vi "仿真全局变量.vi"() -> ()   [LabVIEW 2016, in "仿真数据.lvlib"]
panel:
  in  "关闭":T1(ring)=enum."08"
  in  "开启":T2(ring)=enum."关闭"
  in  "CODMN Reference data in":cluster{"参考数值":dbl[], "参考数值时间戳":timestamp[]}
  in  "CODMN data in":cluster{"数值":dbl, "时间标识":timestamp}
  out "CODMN data out":T3
  in  "CODMN Para":T4 {"切换阈值" format="%#_6f"}
  in  "TN Reference data in":cluster{"参考数值":dbl[], "参考数值时间戳":timestamp[]}
  in  "TN data in":cluster{"数值":dbl, "时间标识":timestamp}
  out "TN data out":T3
  in  "TN Para":T4 {"切换阈值" format="%#_6f"}
  in  "TP Reference data in":cluster{"参考数值":dbl[], "参考数值时间戳":timestamp[]}
  in  "TP data in":cluster{"数值":dbl, "时间标识":timestamp}
  out "TP data out":T3
  in  "TP Para":T4 {"切换阈值" format="%#_6f"}
  in  "NH3N Reference data in":cluster{"参考数值":dbl[], "参考数值时间戳":timestamp[]}
  in  "NH3N data in":cluster{"数值":dbl, "时间标识":timestamp}
  out "NH3N data out":T3
  in  "NH3N Para":T4 {"切换阈值" format="%#_6f"}
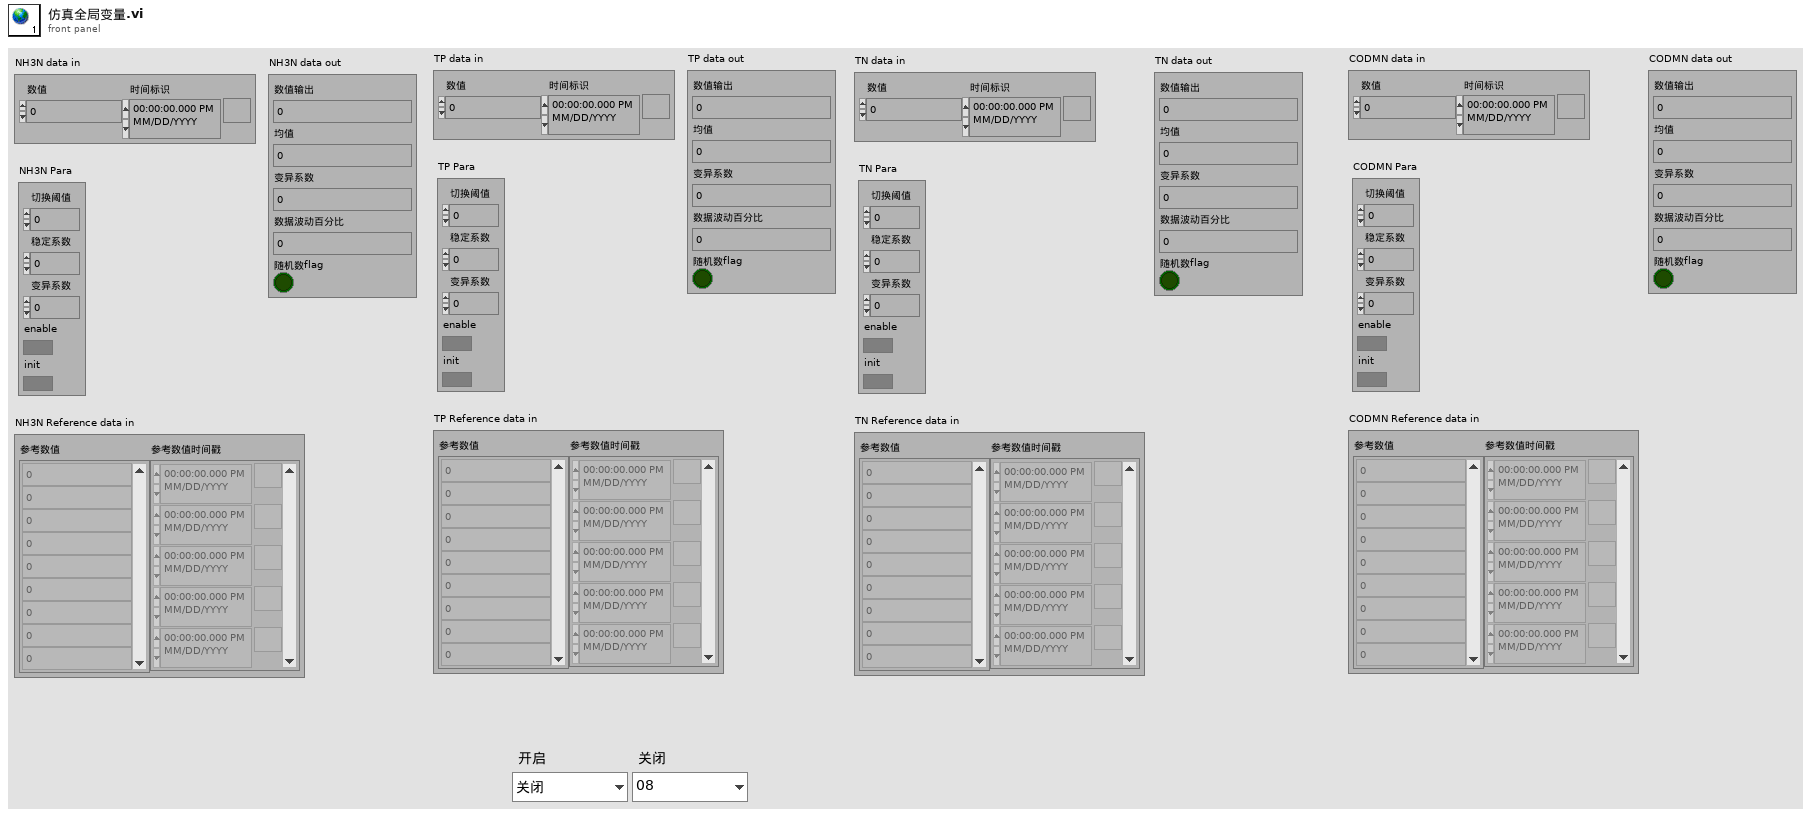
[diagram p1: front panel]
types:
  T1 = enum16{"00", "01", "02", "03", "04", "05", "06", "07", "08", "09", "10", "11", "12", "13", "14", "15", "16", "17", "18", "19", "20", "21", "22", "23"}
  T2 = enum16{"00", "01", "02", "03", "04", "05", "06", "07", "08", "09", "10", "11", "12", "13", "14", "15", "16", "17", "18", "19", "20", "21", "22", "23", "关闭"}
  T3 = cluster{"数值输出":dbl, "均值":dbl, "变异系数":dbl, "数据波动百分比":dbl, "随机数flag":bool}
  T4 = cluster{"切换阈值":dbl, "稳定系数":dbl, "变异系数":dbl, "enable":bool, "init":bool}
diagram:
